vi "DAQmx Create Channel (CI-GPS Timestamp).vi"(0 "task in":refnum<k21>, 1 "gps synchronization method":i32(ring)=10070 items=["IRIG-B"=10070, "PPS"=10080, "None"=10230], 5 "counter":tag, 7 "name to assign":string, 9 "units":i32(ring)=10364 items=["Seconds"=10364, "From Custom Scale"=10065], 11 "error in":errorcluster, 12 "custom scale name":tag) -> (4 "task out":refnum<k21>, 15 "error out":errorcluster)   [LabVIEW 2013]
doc: "Creates a channel that uses a special purpose counter to take a timestamp and synchronizes that counter to a GPS receiver. With the exception of devices that support multi-counter tasks, you can create only one counter input channel at a time with this VI because a task can contain only one counter input channel. To read from multiple counters simultaneously, use a separate task for each counter. Connect the input signals to the default input terminals of the counter unless you select different input terminals."
uses:
  <resource>/objmgr/daqmx.rc
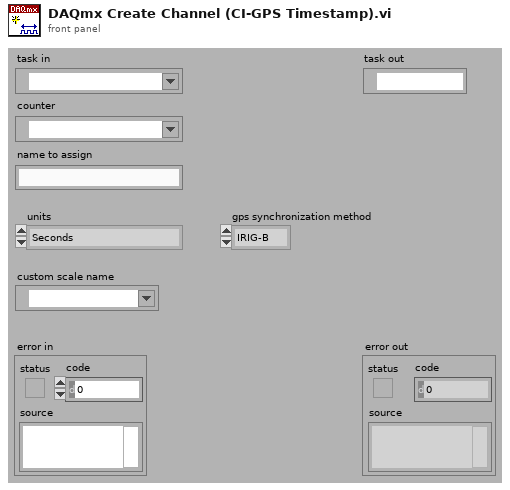
[diagram p1: front panel]
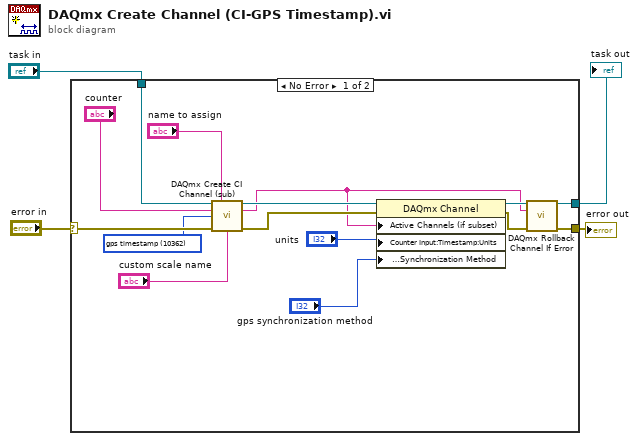
[diagram p0: block diagram]
diagram:
  n1 = case shown="No Error" "error in" {
    selector: "error in" -> [w18 w20]
    tunnel: "task in" -> [w19 w21]
    tunnel: [w12 w21] -> w2
    tunnel: [w10 w20] -> w1
    frame No Error {
      w5 = 10362 items=["count events"=10125, "frequency"=10179, "period"=10256, "pulse width"=10359, "semi period"=10289, "two edge separation"=10267, "angular encoder"=10360, "linear encoder"=10361, "gps timestamp"=10362] ("measurement type")
      n2 = call "DAQmx Create CI Channel (sub).vi"("task in"=w19, "virtual channel name"="name to assign", "physical channel name"="counter", "measurement type"=w5, "error in"=w18, "custom scale"="custom scale name") -> ("task out"=w13:refnum<k21>, "channel names"=w8:string, "error out"=w16:errorcluster)  [unwired: 7 out]
      n3 = property class="DAQmx Channel"(reference=w13, error in=w16, "Active Channels (if subset)"=w8, "Counter Input:Timestamp:Units"="units", "Counter Input:Timestamp:GPS:Synchronization Method"="gps synchronization method") -> (reference out=w11:refnum<k21>, error out=w9:errorcluster)
      n4 = call "DAQmx Rollback Channel If Error.vi"("task in"=w11, "channel names"=w8, "error in"=w9) -> ("task out"=w12:refnum<k21>, "error out"=w10:errorcluster)  [unwired: 11 out]
    }
    frame Error {
    }
  }
  "error out" <- w1
  "task out" <- w2
